vi "4.vi"() -> ()   [LabVIEW 2019]
uses:
  <vilib>/imath/engines/lvmath/Plug In/_Char/NIMS_CH_character datatype.ctl
  <vilib>/imath/engines/lvmath2/RunTimeEngine/Managers/WorkSpace/UID Generator.vi
  <vilib>/imath/engines/lvmath/Plug In/_Char/NIMS_CH_Character RV to String.vi
  <vilib>/imath/engines/lvmath2/RunTimeEngine/BuiltInFunctions/wavread/NIMS_wavread(Str,I32V).vi
  <vilib>/imath/engines/lvmath2/RunTimeEngine/BuiltInFunctions/length/NIMS_length(GM).vi
  <instcachedir>/0/NIMS_length(GM)_47CEC356FCE0482D9BA47DC61C99F2C7.lvgen/NIMS_length(GM)_47CEC356FCE0482D9BA47DC61C99F2C7_000.vi
  <vilib>/imath/engines/lvmath2/RunTimeEngine/BuiltInFunctions/crosscorr/NIMS_crosscorr(GM,GM,Str).vi
  <instcachedir>/0/NIMS_crosscorr(GM,GM,Str)_E2B688A058B24E62B61F0BB8631EA9D6.lvgen/NIMS_crosscorr(GM,GM,Str)_E2B688A058B24E62B61F0BB8631EA9D6_000.vi
  <vilib>/imathl/engines/lvmath/Functions/Error Handling/Create Error.vi
  <vilib>/imath/engines/lvmath2/RunTimeEngine/BuiltInFunctions/max/1 input/NIMS_max(RM).vi
  <instcachedir>/0/NIMS_max(RM)_0B4294876EE440609D638D7C5C6E788E.lvgen/NIMS_max(RM)_0B4294876EE440609D638D7C5C6E788E_000.vi
  <vilib>/imath/engines/lvmath2/RunTimeEngine/BuiltInFunctions/abs/NIMS_abs(signed).vi
  <instcachedir>/0/NIMS_abs(signed)_C4FCB8E6058B49B797C7C8D53CA5F6EC.lvgen/NIMS_abs(signed)_C4FCB8E6058B49B797C7C8D53CA5F6EC_007.vi
  <vilib>/imath/engines/lvmath2/RunTimeSupport/NIMS_Get Scalar_w Error.vi
  <instcachedir>/0/NIMS_Get Scalar_w Error_90FA09EFB1C84794B43793796939E0E3.lvgen/NIMS_Get Scalar_w Error_90FA09EFB1C84794B43793796939E0E3_010.vi
  <vilib>/imath/engines/lvmath2/RunTimeEngine/BuiltInFunctions/crosscorr/NIMS_crosscorr(GM,GM,Sca,Str).vi
  <instcachedir>/0/NIMS_crosscorr(GM,GM,Sca,Str)_61C651AC3D104F16AECC8C9F43556ECD.lvgen/NIMS_crosscorr(GM,GM,Sca,Str)_61C651AC3D104F16AECC8C9F43556ECD_000.vi
  <vilib>/imath/engines/lvmath2/RunTimeEngine/ErrorHandling/NIMS_Create Error From Enums.vi
  <vilib>/imath/engines/lvmath2/RunTimeEngine/IndexRead/NIMS M(R2).vi
  <instcachedir>/0/NIMS M(R2)_287818D58BD74005B29FE73CE7602B1A.lvgen/NIMS M(R2)_287818D58BD74005B29FE73CE7602B1A_000.vi
  <vilib>/imath/engines/lvmath2/RunTimeEngine/BuiltInFunctions/crosscorr/NIMS_crosscorr(GM,Str).vi
  <instcachedir>/0/NIMS_crosscorr(GM,Str)_7E3A3CE9917B451394D0C3CD4C3D6955.lvgen/NIMS_crosscorr(GM,Str)_7E3A3CE9917B451394D0C3CD4C3D6955_000.vi
  <vilib>/imath/engines/lvmath2/RunTimeEngine/BuiltInFunctions/histogram/NIMS_[M]=histogram(M).vi
  <vilib>/imath/engines/lvmath2/RunTimeEngine/BuiltInFunctions/var/NIMS_var(GM,RV).vi
  <instcachedir>/0/NIMS_var(GM,RV)_23A3ACE84EA74C8FB8EF72B06AC4E880.lvgen/NIMS_var(GM,RV)_23A3ACE84EA74C8FB8EF72B06AC4E880_001.vi
  <vilib>/imath/engines/lvmath2/RunTimeEngine/BuiltInFunctions/num_to_str/NIMS_num_to_str(GRowV,I32).vi
  <instcachedir>/0/NIMS_num_to_str(GRowV,I32)_4BA4510D64AF4E68B18295D765365DA3.lvgen/NIMS_num_to_str(GRowV,I32)_4BA4510D64AF4E68B18295D765365DA3_000.vi
  <vilib>/imath/engines/lvmath/Plug In/_Char/NIMS_CH_String to Character Array.vi
  <vilib>/imath/engines/lvmath2/RunTimeEngine/RunTimeType/NIMS_RunTimeType_From StrictType (excl LVString).vi
  <instcachedir>/0/NIMS_RunTimeType_From StrictType (excl LVString)_D8AFBA86A94845AAA577C895450664BD.lvgen/NIMS_RunTimeType_From StrictType (excl LVString)_D8AFBA86A94845AAA577C895450664BD_001.vi
  <vilib>/imath/engines/lvmath2/RunTimeEngine/LocalVariableDefStatement/MC_LocalVariableDefStatement_Display.vi
  <vilib>/imath/engines/lvmath2/RunTimeEngine/BuiltInFunctions/mean/NIMS_RRow=mean(RM,I32).vi
  <vilib>/imath/engines/lvmath2/RunTimeEngine/ErrorHandling/NIMS_Error From Error Code.vi
  <vilib>/imath/engines/lvmath2/RunTimeSupport/NIMS_Get Any Vector_w Error - Matrix.vi
  <instcachedir>/0/NIMS_Get Any Vector_w Error - Matrix_C1DD5EF0FDEC437384B2C8C25171657A.lvgen/NIMS_Get Any Vector_w Error - Matrix_C1DD5EF0FDEC437384B2C8C25171657A_001.vi
  <vilib>/imath/engines/lvmath2/RunTimeEngine/BuiltInFunctions/density_kernel/NIMS_density_kernel(V,Var).vi
  <vilib>/imath/engines/lvmath2/RunTimeEngine/Managers/SymbolTable/Clear UID.vi
  <vilib>/imath/engines/lvmath2/RunTimeEngine/NodeEndStatement/NIMS_NodeEndStatement_Output.vi
  <instcachedir>/0/NIMS_NodeEndStatement_Output_53EC0D466D134D7ABD903AC30B43404B.lvgen/NIMS_NodeEndStatement_Output_53EC0D466D134D7ABD903AC30B43404B_001.vi
  <instcachedir>/0/NIMS_NodeEndStatement_Output_53EC0D466D134D7ABD903AC30B43404B.lvgen/NIMS_NodeEndStatement_Output_53EC0D466D134D7ABD903AC30B43404B_005.vi
  <instcachedir>/0/NIMS_NodeEndStatement_Output_53EC0D466D134D7ABD903AC30B43404B.lvgen/NIMS_NodeEndStatement_Output_53EC0D466D134D7ABD903AC30B43404B_010.vi
  <instcachedir>/0/NIMS_NodeEndStatement_Output_53EC0D466D134D7ABD903AC30B43404B.lvgen/NIMS_NodeEndStatement_Output_53EC0D466D134D7ABD903AC30B43404B_002.vi
  <vilib>/imath/engines/lvmath2/RunTimeEngine/ErrorHandling/NIMS_Finalize Error.vi
  <vilib>/imath/engines/lvmath2/RunTimeEngine/Managers/SymbolTable/NIMS_WorkSpace.lvlib
panel:
  out "频率":dbl
  out "总时间":dbl
  out "延迟时间":dbl[](array[numeric])
  out "延迟点数":dbl[](array[numeric])
  out "概率密度估计":dbl[](graph)
  out "填充信号直方图":i32[][](graph)
  out "填充信号自相关":dbl[][](graph)
  out "填充信号":dbl[][](graph)
  out "放大时间尺度后两路信号自相关":dbl[][](graph)
  out "两路信号自相关":dbl[][](graph)
  out "延时信号":dbl[][](graph)
  out "原始信号":dbl[][](graph)
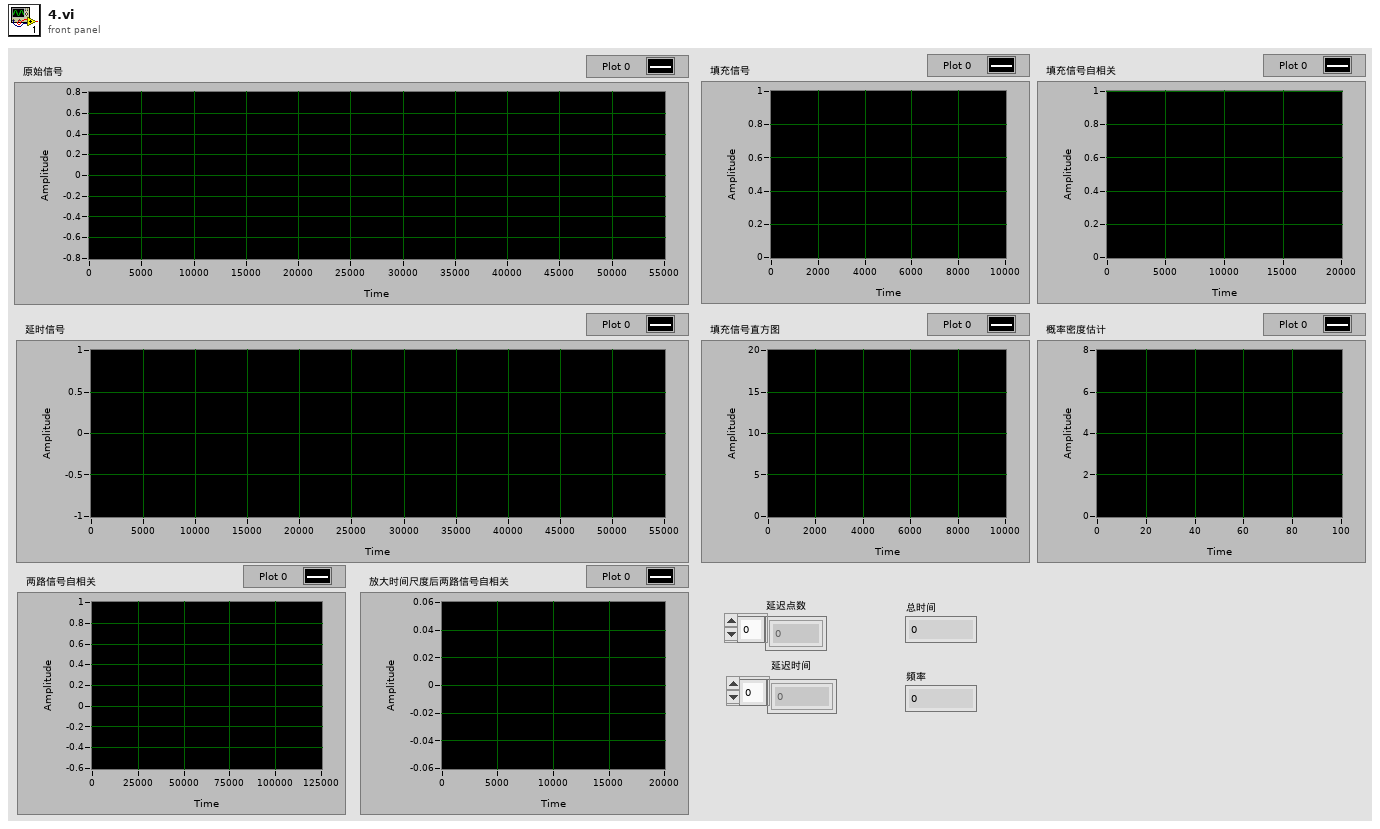
[diagram p1: front panel]
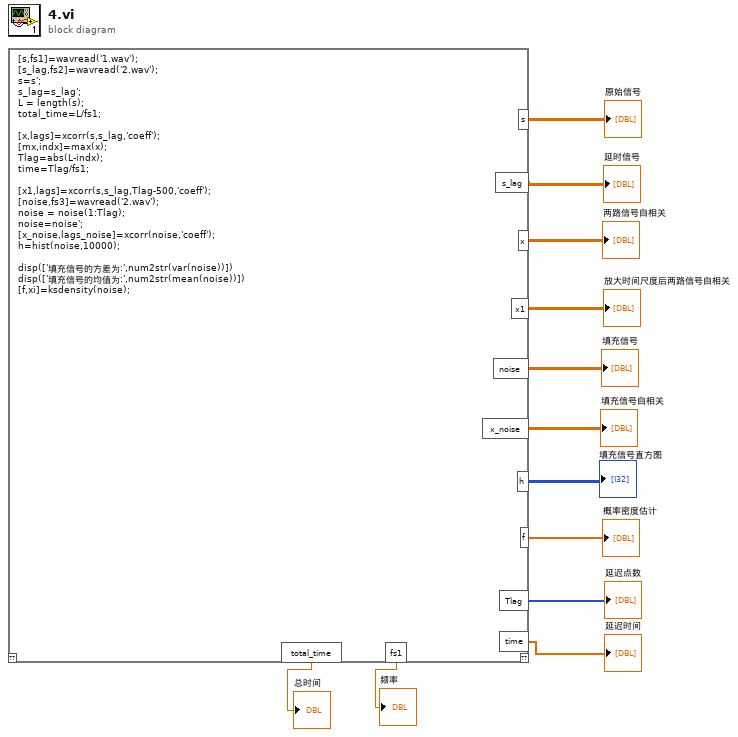
[diagram p0: block diagram]
diagram:
  n1 = mathscript code="[s,fs1]=wavread('1.wav');\n[s_lag,fs2]=wavread('2.wav');\ns=s';\ns_lag=s_lag';\nL = length(s);\ntotal_time=L/fs1;\n\n[x,lags]=xcorr(s,s_lag,'coeff');\n[mx,indx]=max(x);\nTlag=abs(L-indx);\ntime=Tlag/fs1;\n\n[x1,lags]=xcorr(s,s_lag,Tlag-500,'coeff');\n[noise,fs3]=wavread('2.wav');\nnoise = noise(1:Tlag);\nnoise=noise';\n[x_noise,lags_noise]=xcorr(noise,'coeff');\nh=hist(noise,10000);\n\ndisp(['填充信号的方差为:',num2str(var(noise))])\ndisp(['填充信号的均值为:',num2str(mean(noise))])\n[f,xi]=ksdensity(noise);"() -> ("s"=→"原始信号":dbl[][], "s_lag"=→"延时信号":dbl[][], "x"=→"两路信号自相关":dbl[][], "x1"=→"放大时间尺度后两路信号自相关":dbl[][], "noise"=→"填充信号":dbl[][], "x_noise"=→"填充信号自相关":dbl[][], "h"=→"填充信号直方图":i32[][], "f"=→"概率密度估计":dbl[], "Tlag"=→"延迟点数":i32[], "time"=→"延迟时间":dbl[], "fs1"=→"频率":dbl, "total_time"=→"总时间":dbl)  [unwired: 1 in, 1 out]
